vi "Normalized Frame Logic.vi"(11 "Array in":dbl[](array[numeric])) -> (3 "Array out":dbl[](array[numeric]))   [LabVIEW 2012]
doc: "This VI normalizes the control output from the frame to the motors in order to ensure that no in resulting control effort for any motor exceeds the maximum magnitude of 1.\nIf an element is detected to exceed that maximum, all elements within the array are normalized with respect to that maximum.\nIf no element exceeds the maximum, array is left unaltered and pasted through.\nRuffin"
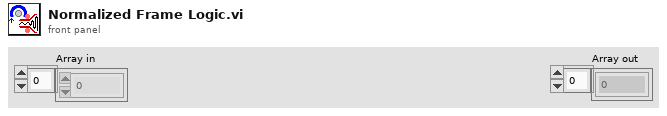
[diagram p1: front panel]
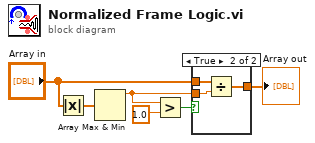
[diagram p0: block diagram]
diagram:
  n1 = Absolute Value(x="Array in") -> (abs(x)=w6:dbl[])
  n2 = Array Max & Min(array=w6) -> (max value=w3:dbl)  [unwired: 3 out]
  n3 = Greater?(x=w3, y=1.0) -> (0:w4:bool)
  n4 = case shown="True" w4 {
    tunnel: "Array in" -> [w7 w10]
    tunnel: w3 -> [_ w9]
    tunnel: [w7 w8] -> w1
    frame False {
    }
    frame True {
      n5 = Divide(x=w10, y=w9) -> (x/y=w8:dbl[])
    }
  }
  "Array out" <- w1
